vi "check RTOS and resend.vi"(8 "error in":errorcluster) -> (0 "error out 2":errorcluster)   [LabVIEW 2016]
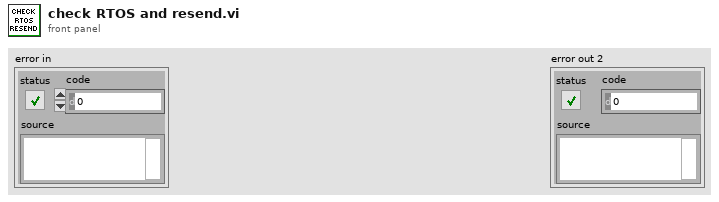
[diagram p1: front panel]
types:
  T1 = cluster{"Hold":bool, "Clamp":bool, "To Set":bool, "To Zero":bool, "Send to IPS":bool, "PS Heat":bool, "Lambda":bool}
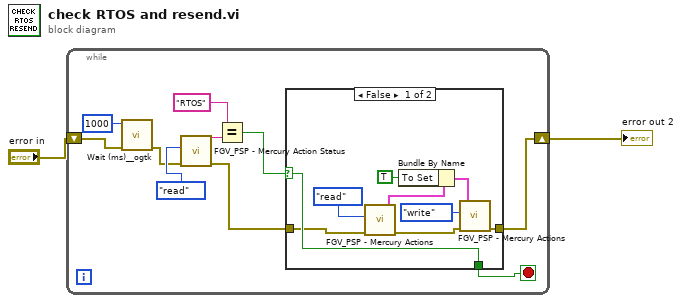
[diagram p0: block diagram]
diagram:
  n1 = while {
    shift-right: [w6] -> w1
    shift-left: "error in" -> [w5]
    stop <- w8 stop-if-true
    n2 = call <userlib>:"Wait (ms)__ogtk.vi"("error in (no error)"=w5, "milliseconds to wait"=u32 1000) -> ("error out"=w4:errorcluster)  [unwired: 8 in, 1 out]
    n3 = call "FGV_PSP - Mercury Action Status.vi"("error in"=w4, "Function"=enum16{"write", "read"}."read") -> ("error out"=w7:errorcluster, "Mercury Status 2"=w12:string)  [unwired: 4 in]
    n4 = Equal?(x="RTOS", y=w12) -> (x = y?=w9:bool)
    n5 = case shown="False" w9 {
      selector: w9 -> [w17 w22]
      tunnel: [w17 w22] -> w8
      tunnel: w7 -> [w15 w23]
      tunnel: [w18 w23] -> w6
      frame False {
        n6 = call "FGV_PSP - Mercury Actions.vi"("error in"=w15, "Function"=enum16{"write", "read"}."read") -> ("error out"=w14:errorcluster, "mercury actions 2"=w13:T1)  [unwired: 4 in]
        n7 = Bundle By Name(cluster=w13, "To Set"=TRUE ("Send to IPS")) -> (w21:T1)
        n8 = call "FGV_PSP - Mercury Actions.vi"("error in"=w14, "Function"=enum16{"write", "read"}."write", "mercury actions"=w21) -> ("error out"=w18:errorcluster)  [unwired: 3 in, 1 out]
      }
      frame True {
      }
    }
  }
  "error out 2" <- w1
